vi "SplitStringIntoArray.vi"(8 "remove empty entries? (F)":bool, 10 "seperators":string="\n", 11 "text":string) -> (2 "number of result strings":i32, 3 "result":string[](array[string]))   [LabVIEW 2011]
panel:
  out "last string len":i32
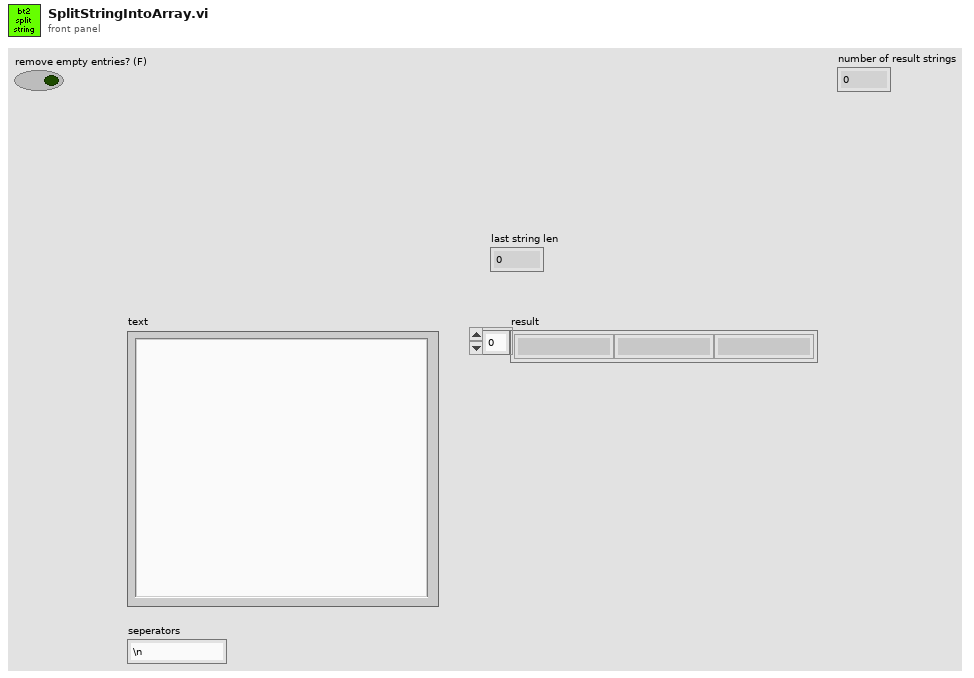
[diagram p1: front panel]
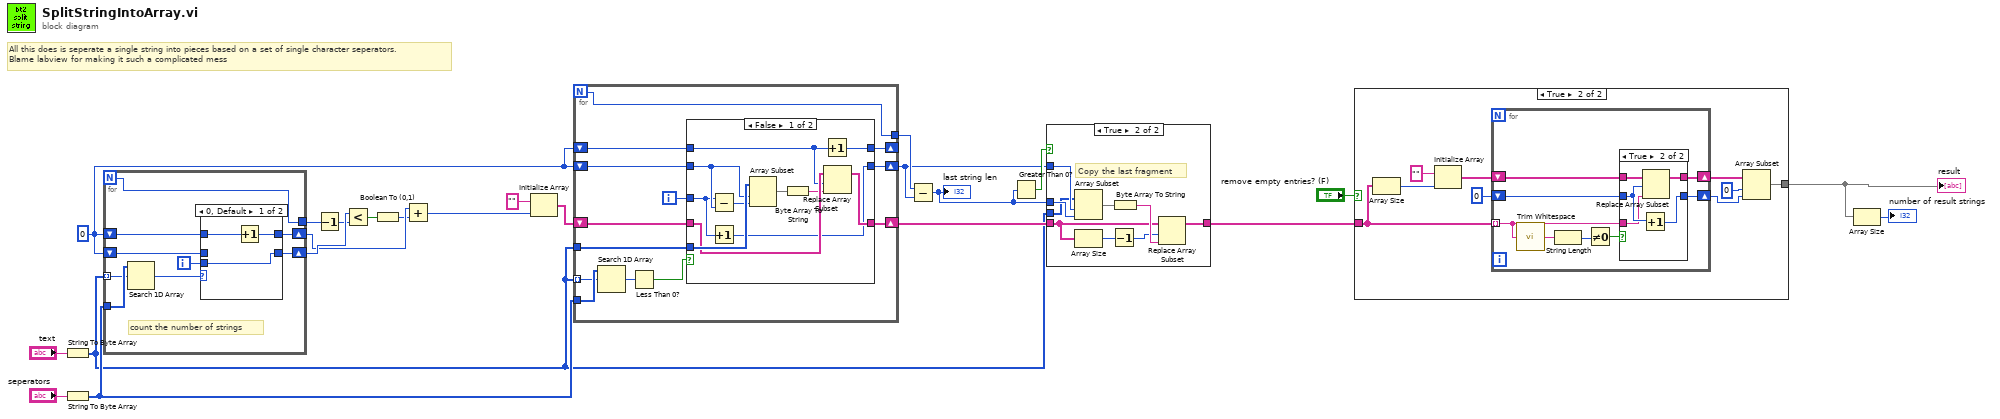
[diagram p0: block diagram]
diagram:
  w18 = 0
  # "All this does is seperate a single string into pieces based on a set of single character seperators.\nBlame labview for making it such a complicated mess"
  n1 = String To Byte Array(string="text") -> (unsigned byte array=w6:u8[])
  n2 = String To Byte Array(string="seperators") -> (unsigned byte array=w19:u8[])
  n3 = for {
    N -> [w24]
    tunnel: w6 -> [w29] mode=indexing
    shift-right: [w32] -> w13
    shift-left: w18 -> [w31]
    tunnel: w19 -> [w30]
    shift-right: [w25] -> w17
    shift-left: w18 -> [w27]
    tunnel: [w24] -> w16
    i -> [w26]
    # "count the number of strings"
    n4 = Search 1D Array(1D array=w30, element=w29) -> (index of element=w28:i32)  [unwired: 1 in]
    n5 = case shown="0, Default" w28 {
      tunnel: [w34 w37] -> w32
      tunnel: w31 -> [w35 w37]
      tunnel: w27 -> [_ w36]
      tunnel: w26 -> [w33 _]
      tunnel: [w33 w36] -> w25
      frame 0, Default {
        n6 = Increment(x=w35) -> (x+1=w34:i32)
      }
      frame -1 {
      }
    }
  }
  n7 = Decrement(x=w16) -> (x-1=w15:i32)
  n8 = Less?(x=w17, y=w15) -> (x < y?=w14:bool)
  n9 = Boolean To (0,1)(Boolean=w14) -> (0, 1=w12:i16)
  n10 = Add(x=w13, y=w12) -> (x+y=w11:i32)
  n11 = Initialize Array("" ("String"), w11) -> (w23:string[])
  n12 = for {
    N -> [w38]
    tunnel: w6 -> [w41] mode=indexing
    shift-right: [w50] -> w5
    shift-left: w18 -> [w48]
    tunnel: w6 -> [w47]
    shift-right: [w43] -> _
    shift-left: w18 -> [w46]
    shift-right: [w44] -> w10
    shift-left: w23 -> [w45]
    tunnel: w19 -> [w42]
    tunnel: [w38] -> w9
    i -> [w49]
    n13 = Search 1D Array(1D array=w42, element=w41) -> (index of element=w40:i32)  [unwired: 1 in]
    n14 = Less Than 0?(x=w40) -> (x < 0?=w39:bool)
    n15 = case shown="False" w39 {
      tunnel: [w51 w64] -> w50
      tunnel: w49 -> [w52 _]
      tunnel: w48 -> [w54 w64]
      tunnel: w47 -> [w61 _]
      tunnel: w46 -> [w57 w62]
      tunnel: w45 -> [w59 w63]
      tunnel: [w58 w63] -> w44
      tunnel: [w55 w62] -> w43
      frame False {
        n16 = Subtract(x=w52, y=w54) -> (x-y=w53:i32)
        n17 = Increment(x=w52) -> (x+1=w51:i32)
        n18 = Array Subset(array=w61, index=w54, length=w53) -> (w60:u8[])
        n19 = Byte Array To String(unsigned byte array=w60) -> (string=w56:string)
        n20 = Increment(x=w57) -> (x+1=w55:i32)
        n21 = Replace Array Subset(array=w59, new element=w56, index=w57) -> (w58:string[])
      }
      frame True {
      }
    }
  }
  n22 = Subtract(x=w9, y=w5) -> (x-y=w7:i32)
  "last string len" <- w7
  n23 = Greater Than 0?(x=w7) -> (x > 0?=w8:bool)
  n24 = case shown="True" w8 {
    tunnel: w10 -> [w65 w68]
    tunnel: [w65 w71] -> w3
    tunnel: w5 -> [_ w74]
    tunnel: w7 -> [_ w73]
    tunnel: w6 -> [_ w72]
    frame False {
    }
    frame True {
      # "Copy the last fragment"
      n25 = Array Subset(array=w72, index=w74, length=w73) -> (w70:u8[])
      n26 = Array Size(array=w68) -> (size(s)=w67:i32)
      n27 = Decrement(x=w67) -> (x-1=w66:i32)
      n28 = Byte Array To String(unsigned byte array=w70) -> (string=w69:string)
      n29 = Replace Array Subset(array=w68, new element=w69, index=w66) -> (w71:string[])
    }
  }
  n30 = case shown="True" "remove empty entries? (F)" {
    tunnel: w3 -> [w75 w76]
    tunnel: [w75 w77] -> w2
    frame False {
    }
    frame True {
      n31 = Array Size(array=w76) -> (size(s)=w83:i32)
      n32 = Initialize Array("" ("element"), w83) -> (w81:string[])
      n33 = for {
        tunnel: w76 -> [w85] mode=indexing
        shift-right: [w86] -> w78
        shift-left: 0 -> [w87]
        shift-right: [w88] -> w80
        shift-left: w81 -> [w89]
        n34 = call <vilib>:"Trim Whitespace.vi"("string"=w85) -> ("trimmed string"=w92:string)  [unwired: 1 in]
        n35 = String Length(string=w92) -> (length=w91:i32)
        n36 = Not Equal To 0?(x=w91) -> (x != 0?=w90:bool)
        n37 = case shown="True" w90 {
          tunnel: w89 -> [w94 w99]
          tunnel: [w94 w96] -> w88
          tunnel: w87 -> [w93 w98]
          tunnel: [w93 w97] -> w86
          tunnel: w85 -> [_ w95]
          frame False {
          }
          frame True {
            n38 = Increment(x=w98) -> (x+1=w97:i32)
            n39 = Replace Array Subset(array=w99, new element=w95, index=w98) -> (w96:string[])
          }
        }
      }
      n40 = Array Subset(array=w80, index=0, length=w78) -> (w77:string[])
    }
  }
  "result" <- w2
  n41 = Array Size(array=w2) -> (size(s)=→"number of result strings":i32)
